vi "StringToDBL.vi"(0 "String":string, 7 "Offset":i32 caption="Offset (0)", 11 "Error in":errorcluster caption="Error in (no error)") -> (4 "Number":dbl, 8 "Offset Past Number":i32, 15 "Error out":errorcluster)   [LabVIEW 2017, in "GPString.lvlib"]
doc: "Converts <B>String</B> to <B>Number</B>, starting the conversion from the optional <B>Offset</B> in <B>String</B>.\n\nBoth period (.) and comma (,) are supported as radix point in <B>String</B>.\n\nThis VI is inlined.\n\nSteen Schmidt\nGPower\n23/9 2015"
uses:
  GPString.lvlib
panel:
  # "Copyright © 2016\nGPower\nSee enclosed license file for terms and conditions"
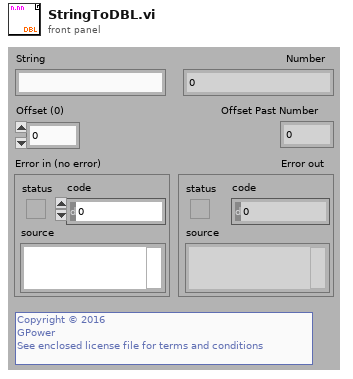
[diagram p1: front panel]
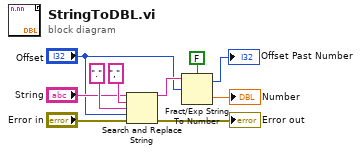
[diagram p0: block diagram]
diagram:
  n1 = Search and Replace String(input string="String", search string=",", replace string="." ("search string"), offset="Offset", error in="Error in") -> (result string=w6:string, error out=→"Error out":errorcluster)  [unwired: 3 in, 2 out]
  n2 = Fract/Exp String To Number(use system decimal point (T)=FALSE, string=w6, offset="Offset") -> (offset past number=→"Offset Past Number":i32, number=→"Number":dbl)  [unwired: 1 in]
